vi "GetPowerSupplyDataField.vi"(10 "Telemetry Data":string, 11 "Cluster in":refnum<vi>) -> (3 "Array":string[](array[string]))   [LabVIEW 2016]
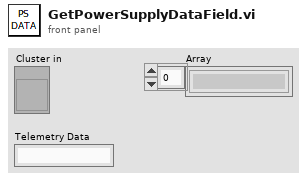
[diagram p1: front panel]
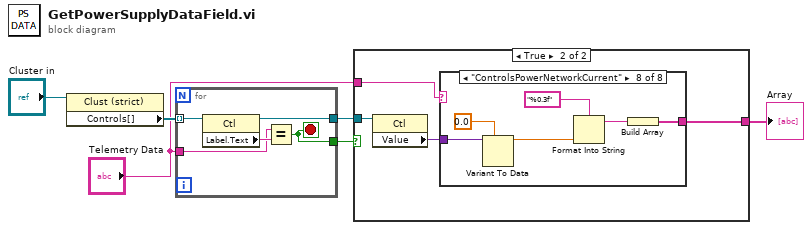
[diagram p0: block diagram]
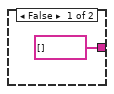
[diagram p2: hidden frame]
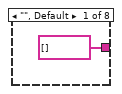
[diagram p3: hidden frame]
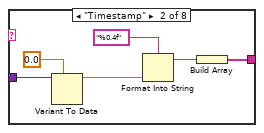
[diagram p4: hidden frame]
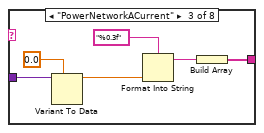
[diagram p5: hidden frame]
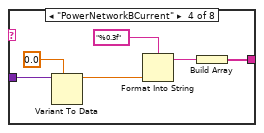
[diagram p6: hidden frame]
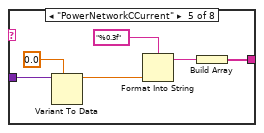
[diagram p7: hidden frame]
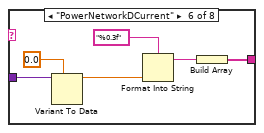
[diagram p8: hidden frame]
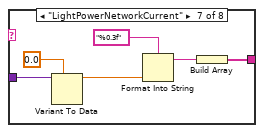
[diagram p9: hidden frame]
diagram:
  n1 = property on="Property Node" class="Clust (strict)"(reference="Cluster in") -> ("Controls[]"=w5:refnum<vi>[])  [unwired: 1 in, 2 out]
  n2 = for {
    tunnel: w5 -> [w11] mode=indexing
    tunnel: [w10] -> w2
    tunnel: "Telemetry Data" -> [w8]
    tunnel: [w7] -> w1
    stop <- w7 stop-if-true
    n3 = property on="Property Node" class="Ctl"(reference=w11) -> (reference out=w10:refnum<vi>, "Label.Text"=w9:string)  [unwired: 1 in, 1 out]
    n4 = Equal?(x=w8, y=w9) -> (x = y?=w7:bool)
  }
  n5 = case shown="True" w1 {
    tunnel: "Telemetry Data" -> [_ w16]
    tunnel: w2 -> [_ w15]
    tunnel: [string[] [] w13] -> w6
    frame False {
    }
    frame True {
      n6 = property on="Property Node" class="Ctl"(reference=w15) -> ("Value"=w14:variant)  [unwired: 1 in, 2 out]
      n7 = case shown="\"ControlsPowerNetworkCurrent\"" w16 {
        tunnel: [string[] [] w21 w27 w33 w39 w45 w51 w57] -> w13
        tunnel: w14 -> [_ w19 w25 w31 w37 w43 w49 w55]
        frame "", Default {
        }
        frame "Timestamp" {
          n8 = Variant To Data(type=0.0, Variant=w19) -> (data=w20:dbl)  [unwired: 1 in, 1 out]
          n9 = Format Into String(format string="%0.4f", w20) -> (resulting string=w22:string)  [unwired: 2 in, 1 out]
          n10 = Build Array(w22) -> (w21:string[])
        }
        frame "PowerNetworkACurrent" {
          n11 = Variant To Data(type=0.0, Variant=w25) -> (data=w26:dbl)  [unwired: 1 in, 1 out]
          n12 = Format Into String(format string="%0.3f", w26) -> (resulting string=w28:string)  [unwired: 2 in, 1 out]
          n13 = Build Array(w28) -> (w27:string[])
        }
        frame "PowerNetworkBCurrent" {
          n14 = Variant To Data(type=0.0, Variant=w31) -> (data=w32:dbl)  [unwired: 1 in, 1 out]
          n15 = Format Into String(format string="%0.3f", w32) -> (resulting string=w34:string)  [unwired: 2 in, 1 out]
          n16 = Build Array(w34) -> (w33:string[])
        }
        frame "PowerNetworkCCurrent" {
          n17 = Variant To Data(type=0.0, Variant=w37) -> (data=w38:dbl)  [unwired: 1 in, 1 out]
          n18 = Format Into String(format string="%0.3f", w38) -> (resulting string=w40:string)  [unwired: 2 in, 1 out]
          n19 = Build Array(w40) -> (w39:string[])
        }
        frame "PowerNetworkDCurrent" {
          n20 = Variant To Data(type=0.0, Variant=w43) -> (data=w44:dbl)  [unwired: 1 in, 1 out]
          n21 = Format Into String(format string="%0.3f", w44) -> (resulting string=w46:string)  [unwired: 2 in, 1 out]
          n22 = Build Array(w46) -> (w45:string[])
        }
        frame "LightPowerNetworkCurrent" {
          n23 = Variant To Data(type=0.0, Variant=w49) -> (data=w50:dbl)  [unwired: 1 in, 1 out]
          n24 = Format Into String(format string="%0.3f", w50) -> (resulting string=w52:string)  [unwired: 2 in, 1 out]
          n25 = Build Array(w52) -> (w51:string[])
        }
        frame "ControlsPowerNetworkCurrent" {
          n26 = Variant To Data(type=0.0, Variant=w55) -> (data=w56:dbl)  [unwired: 1 in, 1 out]
          n27 = Format Into String(format string="%0.3f", w56) -> (resulting string=w58:string)  [unwired: 2 in, 1 out]
          n28 = Build Array(w58) -> (w57:string[])
        }
      }
    }
  }
  "Array" <- w6
